vi "enableOut.vi"(8 "error in (no error)":errorcluster) -> (0 "error out":errorcluster)   [LabVIEW 2019, in "DS360_GPIB.lvlib"]
uses:
  DS360_GPIB.lvlib
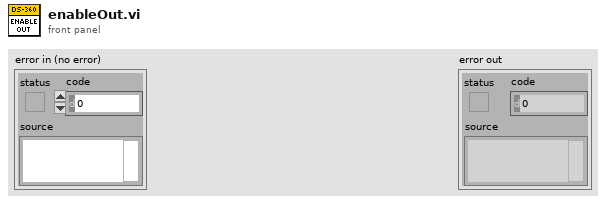
[diagram p1: front panel]
types:
  T1 = cluster{"error":bool, "code":i32, "source":string}
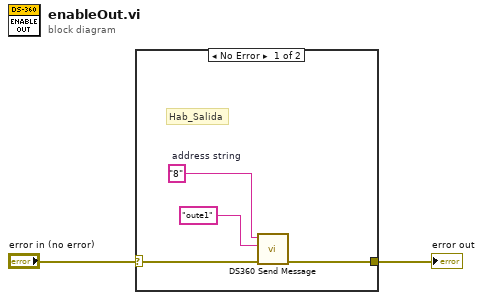
[diagram p0: block diagram]
diagram:
  n1 = case shown="No Error" "error in (no error)" {
    selector: "error in (no error)" -> [w4 w7]
    tunnel: [w3 w7] -> w1
    frame No Error {
      w5 = "8"  # address string
      # "Hab_Salida"
      n2 = call <instrlib>:"DS360 Send Message.vi"("address string"=w5, "write buffer"="oute1", "error in"=w4) -> ("error out"=w3:T1)  [unwired: 3 in, 3 out]
    }
    frame Error {
    }
  }
  "error out" <- w1
